vi "Write Text.vi"(8 "error in (no error)":errorcluster, 10 "Text":string, 11 "FSM.Label in":refnum<class "FSM.Label.lvclass">) -> (0 "error out":errorcluster, 3 "FSM.Label out":refnum<class "FSM.Label.lvclass">)   [LabVIEW 2020, in "FSM.Label.lvclass"]
uses:
  FSM.Label.lvclass
  FSM.Label.lvclass/FSM.Label.ctl
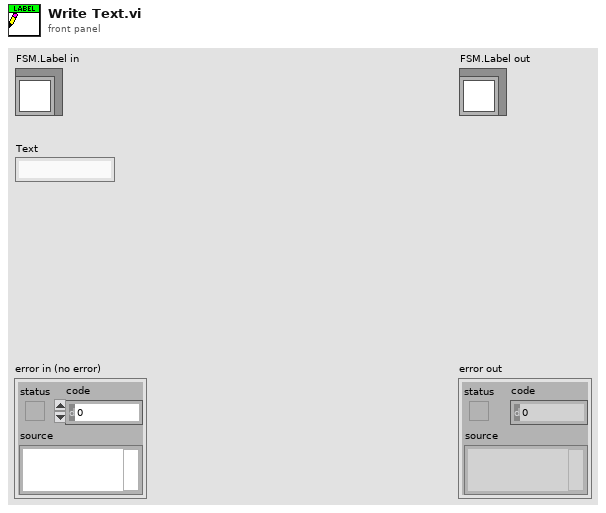
[diagram p1: front panel]
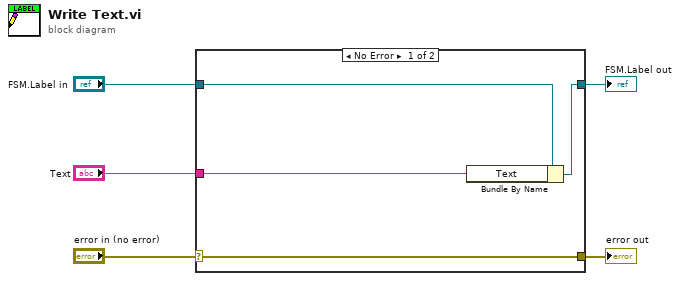
[diagram p0: block diagram]
diagram:
  n1 = case shown="No Error" "error in (no error)" {
    selector: "error in (no error)" -> [w9 w10]
    tunnel: [w9 w10] -> w4
    tunnel: [w7 w11] -> w2
    tunnel: "FSM.Label in" -> [w8 w11]
    tunnel: "Text" -> [w6 _]
    frame No Error {
      n2 = Bundle By Name(cluster=w8, "Text"=w6) -> (w7:refnum<class "FSM.Label.lvclass">)
    }
    frame Error {
    }
  }
  "error out" <- w4
  "FSM.Label out" <- w2
